vi "QMH_Label Localization.vi"() -> (2 "localized control labels":string[](array[string]), 3 "DNL_unlocalized control labels":string[](array[string]), 4 "DNL_unlocalized string constant labels":string[](array[string]), 6 "localized string constant values":string[](array[string]))   [LabVIEW 2018]
doc: "Specifies the labels of the block diagram string constants in the QMH template that contain text that needs to be localized."
panel:
  in  "static localized string constant values":string[](array[string])=["\"Exit\" button pressed", "Initial Message", "\"Do Something\" button pressed", "\"Do Something Else\" button pressed", "The invalid message string \"%s\" was received in the Message Handling Loop."]
  in  "static localized control labels":string[](array[string])
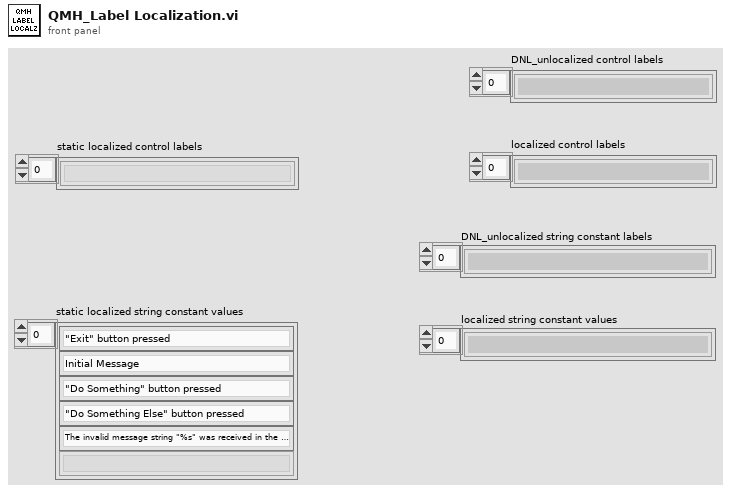
[diagram p1: front panel]
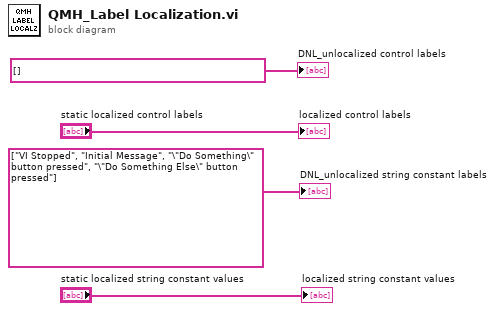
[diagram p0: block diagram]
diagram:
  "DNL_unlocalized control labels" <- string[] [] ("DNL_unlocalized control labels")
  "localized control labels" <- "static localized control labels"
  "localized string constant values" <- "static localized string constant values"
  "DNL_unlocalized string constant labels" <- string[] ["VI Stopped", "Initial Message", "\"Do Something\" button pressed", "\"Do Something Else\" button pressed"] ("DNL_unlocalized control labels")
